vi "Get Local Chassis All Slots References.vi"(8 "error in":errorcluster, 11 "Local Chassis Reference In":T1 format="%.0x") -> (0 "error out":errorcluster, 1 "Modules Found":bool, 2 "Slots References":T1[](array[typedef]) format="%.0x", 3 "Local Chassis Reference Out":T1 format="%.0x")   [LabVIEW 2019, in "SEECD System Explorer.lvlib"]
uses:
  SEECD System Explorer.lvlib
  <vilib>/NI VeriStand/Custom Device Tools/Custom Device Utility Library/Custom Device Utility Library.lvlib
  Shared/Globals/Scan Engine GUIDs.vi
  Shared/SEECD Shared.lvlib
  Includes/Modules.lvlibp/RSI Module/RSI Module.lvclass
  <vilib>/NI VeriStand/Custom Device Tools/Custom Device Utility Library/NI VeriStand - Search for All Items by GUID.vi
  <vilib>/NI VeriStand/Custom Device API/Custom Device Item Ref.ctl
  <vilib>/NI VeriStand/Custom Device API/Custom Device API.lvlib
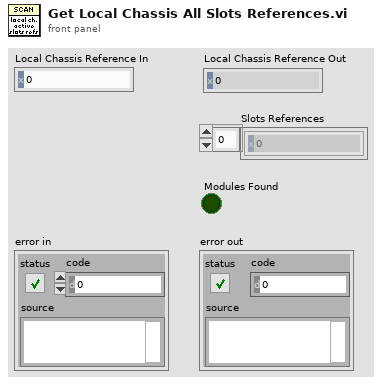
[diagram p1: front panel]
types:
  T1 = typedef "Custom Device API.lvlib/Custom Device Item Ref.ctl" = u64
  T2 = typedef "Modules.lvlibp/Custom Device API.lvlib/Custom Device Item Ref.ctl" = u64
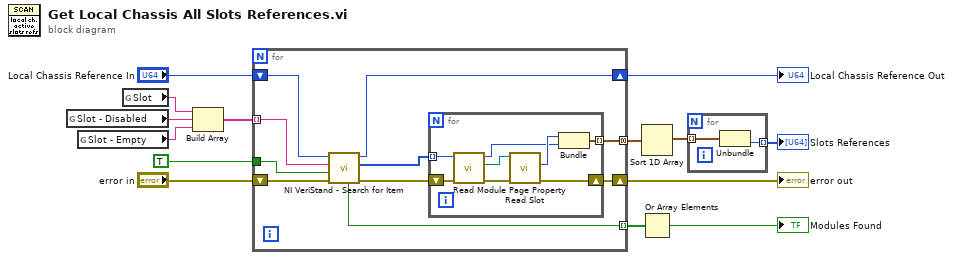
[diagram p0: block diagram]
diagram:
  n1 = global read "Scan Engine GUIDs.vi" "Slot - Disabled"() -> (w5:string)
  n2 = global read "Scan Engine GUIDs.vi" "Slot - Empty"() -> (w4:string)
  n3 = global read "Scan Engine GUIDs.vi" "Slot"() -> (w14:string)
  n4 = Build Array(w14, w5, w4) -> (w6:string[])
  n5 = for {
    tunnel: w6 -> [w24] mode=indexing
    shift-right: [w20] -> w8
    shift-left: "Local Chassis Reference In" -> [w22]
    shift-right: [w18] -> w13
    shift-left: "error in" -> [w21]
    tunnel: TRUE ("Find All? (T)") -> [w23]
    tunnel: [w17] -> w12 mode=indexing
    tunnel: [w15] -> w3 mode=concatenating
    n6 = call-poly <vilib>:"NI VeriStand - Search for Item.vi"("error in"=w21, "Find All? (T)"=w23, "Item GUID"=w24, "Section Ref in"=w22) -> ("error out"=w19:errorcluster, "Item Refs"=w16:T1[], "Section Ref out"=w20:T1, "Found"=w17:bool)  [unwired: 4 in]
    n7 = for {
      shift-right: [w31] -> w18
      shift-left: w19 -> [w32]
      tunnel: w16 -> [w27] mode=indexing
      tunnel: [w25] -> w15 mode=indexing
      n8 = call "Read Module Page Property.vi"("error in (no error)"=w32, "Node Ptr In"=w27) -> ("error out"=w30:errorcluster, "RSI Module"=w29:refnum<class "RSI Module.lvclass">, "Node Ptr Out"=w26:T2)  [unwired: 7 in]
      n9 = call "Read Slot.vi"("error in (no error)"=w30, "RSI Module in"=w29) -> ("error out"=w31:errorcluster, "Slot"=w28:u32)  [unwired: 7 in, 1 out]
      n10 = Bundle("Slot"=w28, "Node Ptr Out"=w26) -> (w25:cluster{"Slot":u32, "Node Ptr Out":T2})  [unwired: 1 in]
    }
  }
  "error out" <- w13
  "Local Chassis Reference Out" <- w8
  n11 = Sort 1D Array(array=w3) -> (sorted array=w2:cluster{"Slot":u32, "Node Ptr Out":T2}[])
  n12 = Or Array Elements(Boolean array=w12) -> (logical OR=→"Modules Found":bool)
  n13 = for {
    tunnel: w2 -> [w34] mode=indexing
    tunnel: [w33] -> w1 mode=indexing
    n14 = Unbundle(w34) -> ("Node Ptr Out"=w33:T2)  [unwired: 1 out]
  }
  "Slots References" <- w1
